vi "Main.vi"(8 "error in (no error)":errorcluster, 11 "FactoryMethodDemo":refnum<class "FactoryMethodDemo.lvclass">) -> (0 "error out":errorcluster, 3 "FactoryMethodDemo":refnum<class "FactoryMethodDemo.lvclass">)   [LabVIEW 2020, in "FactoryMethod.lvlib" / "FactoryMethodDemo.lvclass"]
uses:
  FactoryMethodDemo.lvclass
  Support/Lib/HSE-Logger/LogLevel.ctl
  ConcreteCreatorA/ConcreteCreatorA.lvclass
  E:/GitHub/Design-Patterns-GoF_-_NI-LV/Creational/FactoryMethod/Base_Example/Creator/Creator.lvclass
  ConcreteCreatorB/ConcreteCreatorB.lvclass
  Support/Class/ConsoleOutput.lvclass
  Support/Lib/hse-logger.lvlib
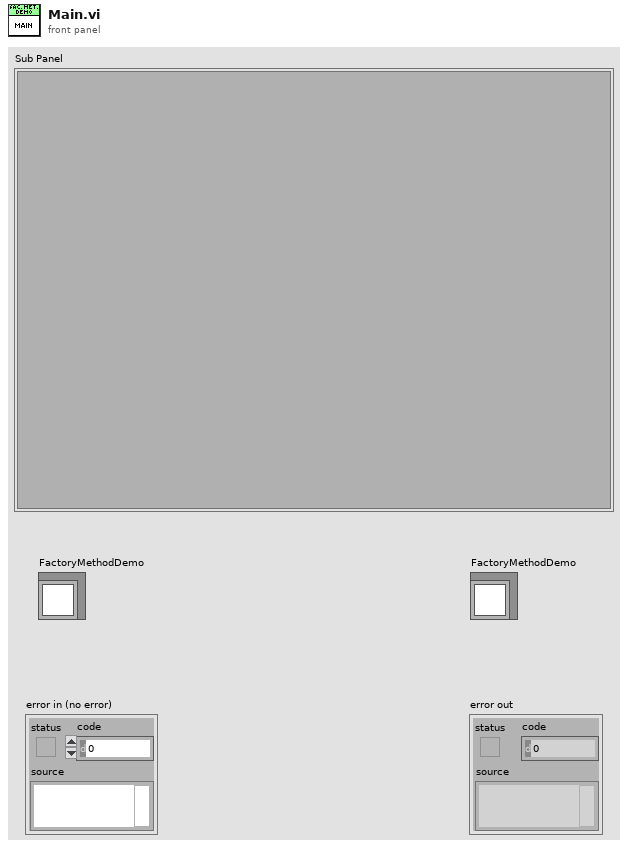
[diagram p1: front panel]
types:
  T1 = typedef "hse-logger.lvlib/LogLevel.ctl" = enum16{"DEBUG", "INFO", "WARNING", "ERROR", "CRITICAL"}
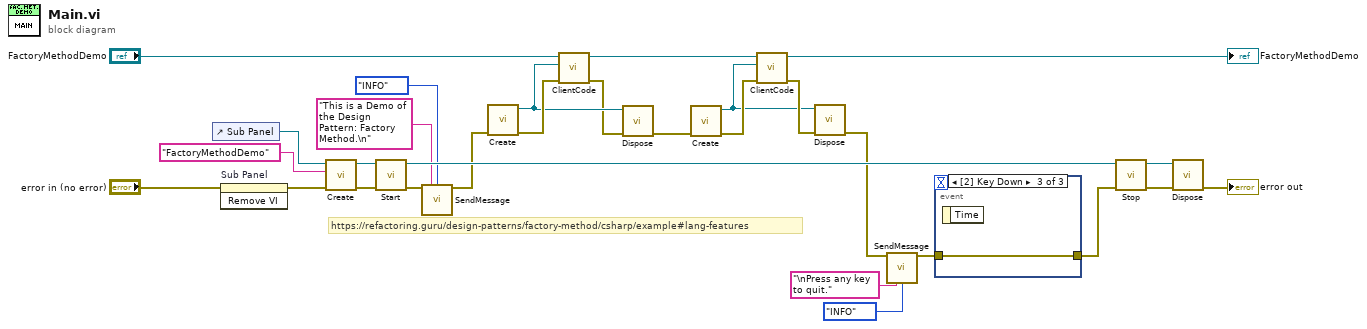
[diagram p0: block diagram]
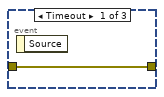
[diagram p2: hidden frame]
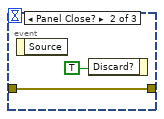
[diagram p3: hidden frame]
diagram:
  # "https://refactoring.guru/design-patterns/factory-method/csharp/example#lang-features"
  n1 = control-ref of="Sub Panel"() -> (w7:refnum<vi>)
  n2 = invoke on="Sub Panel" class="SubPnl" method="Remove VI"(error in="error in (no error)") -> (error out=w8:errorcluster)  [unwired: 2 in, 2 out]
  n3 = call "Create.vi"("error in (no error)"=w8, "LoggerName"="FactoryMethodDemo", "SubPanelRef"=w7) -> ("error out"=w29:errorcluster, "ConsoleOutput out"=w28:refnum<class "ConsoleOutput.lvclass">)  [unwired: 7 in]
  n4 = call "Start.vi"("error in (no error)"=w29, "ConsoleOutput in"=w28) -> ("error out"=w21:errorcluster, "ConsoleOutput out"=w24:refnum<class "ConsoleOutput.lvclass">)  [unwired: 8 in]
  n5 = call "SendMessage.vi"("Level"=LogLevel."INFO", "Message"="This is a Demo of the Design Pattern: Factory Method.\n" ("Data"), "error in (no error)"=w21) -> ("error out"=w19:errorcluster)  [unwired: 12 in]
  n6 = call "Create.vi"("error in (no error)"=w19) -> ("error out"=w18:errorcluster, "ConcreteCreatorA out"=w13:refnum<class "ConcreteCreatorA.lvclass">)  [unwired: 9 in]
  n7 = call "ClientCode.vi"("error in (no error)"=w18, "Creator"=w13, "FactoryMethodDemo in"="FactoryMethodDemo") -> ("error out"=w12:errorcluster, "FactoryMethodDemo out"=w15:refnum<class "FactoryMethodDemo.lvclass">)  [unwired: 7 in]
  n8 = call-dynamic "Dispose.vi"("error in (no error)"=w12, "ConcreteCreatorA in"=w13) -> ("error out"=w5:errorcluster)  [unwired: 9 in]
  n9 = call "Create.vi"("error in (no error)"=w5) -> ("error out"=w14:errorcluster, "ConcreteCreatorA out"=w10:refnum<class "ConcreteCreatorB.lvclass">)  [unwired: 9 in]
  n10 = call "ClientCode.vi"("error in (no error)"=w14, "Creator"=w10, "FactoryMethodDemo in"=w15) -> ("error out"=w11:errorcluster, "FactoryMethodDemo out"=→"FactoryMethodDemo":refnum<class "FactoryMethodDemo.lvclass">)  [unwired: 7 in]
  n11 = call-dynamic "Dispose.vi"("error in (no error)"=w11, "ConcreteCreatorA in"=w10) -> ("error out"=w3:errorcluster)  [unwired: 9 in]
  n12 = call "SendMessage.vi"("Level"=LogLevel."INFO", "Message"="\nPress any key to quit." ("Data"), "error in (no error)"=w3) -> ("error out"=w4:errorcluster)  [unwired: 12 in]
  n13 = event shown="[2] Key Down" {
    selector: _ -> [_ _ _]
    dyn-events: _ -> [_ _ _]
    timeout: _ -> [_ _ _]
    tunnel: w4 -> [w30 w32 w33]
    tunnel: [w30 w32 w33] -> w22
    event Timeout {
      n14 = event-data() -> ()  [unwired: 1 in, 1 out]
    }
    event Panel Close? {
      n15 = event-data() -> ()  [unwired: 1 in, 1 out]
      n16 = event-data("Discard?"=TRUE) -> ()  [unwired: 1 in, 1 out]
    }
    event Key Down {
      n17 = event-data() -> ()  [unwired: 1 in, 1 out]
    }
  }
  n18 = call "Stop.vi"("error in (no error)"=w22, "ConsoleOutput in"=w24) -> ("error out"=w26:errorcluster, "ConsoleOutput out"=w25:refnum<class "ConsoleOutput.lvclass">)  [unwired: 8 in]
  n19 = call "Dispose.vi"("error in (no error)"=w26, "ConsoleOutput in"=w25) -> ("error out"=→"error out":errorcluster)  [unwired: 9 in]
